vi "generate_simulated_signals.vi"() -> ()   [LabVIEW 2013]
panel:
  out "Mixer signal":dbl[](graph)
  out "Simulated":i16[](graph)
  out "Sine out":fxp<+/-,16,0>[][](array[numeric])
  out "Cosine out":fxp<+/-,16,0>[][](array[numeric])
  out "simulated 2D":i16[][](array[numeric])
  out "simulated 1D":i16[](array[numeric])
  out "sin":fxp<+/-,16,0>[](array[numeric])
  out "cos":fxp<+/-,16,0>[](array[numeric])
  out "Numeric":i32
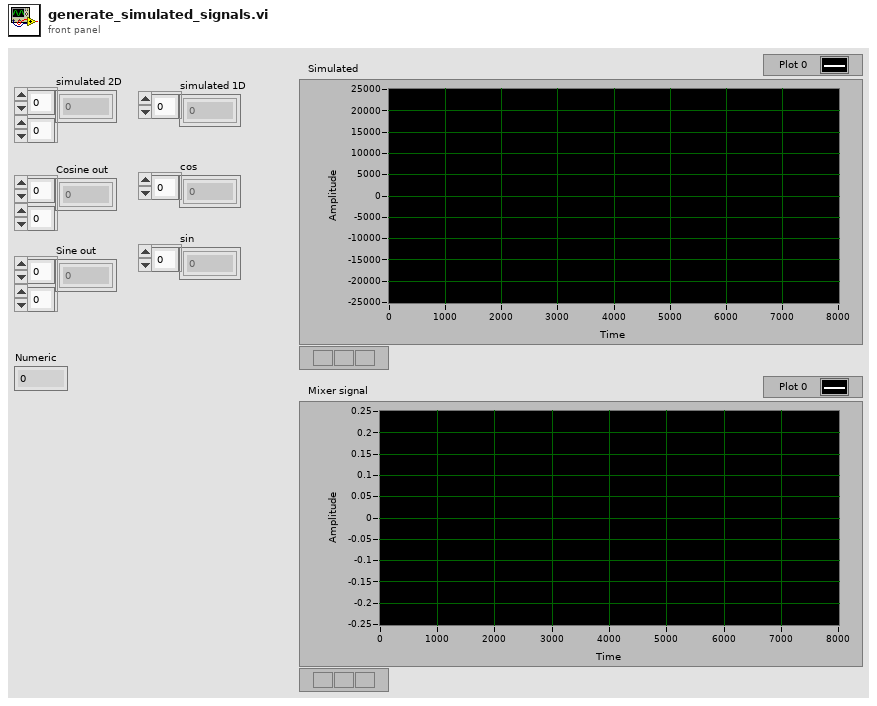
[diagram p1: front panel]
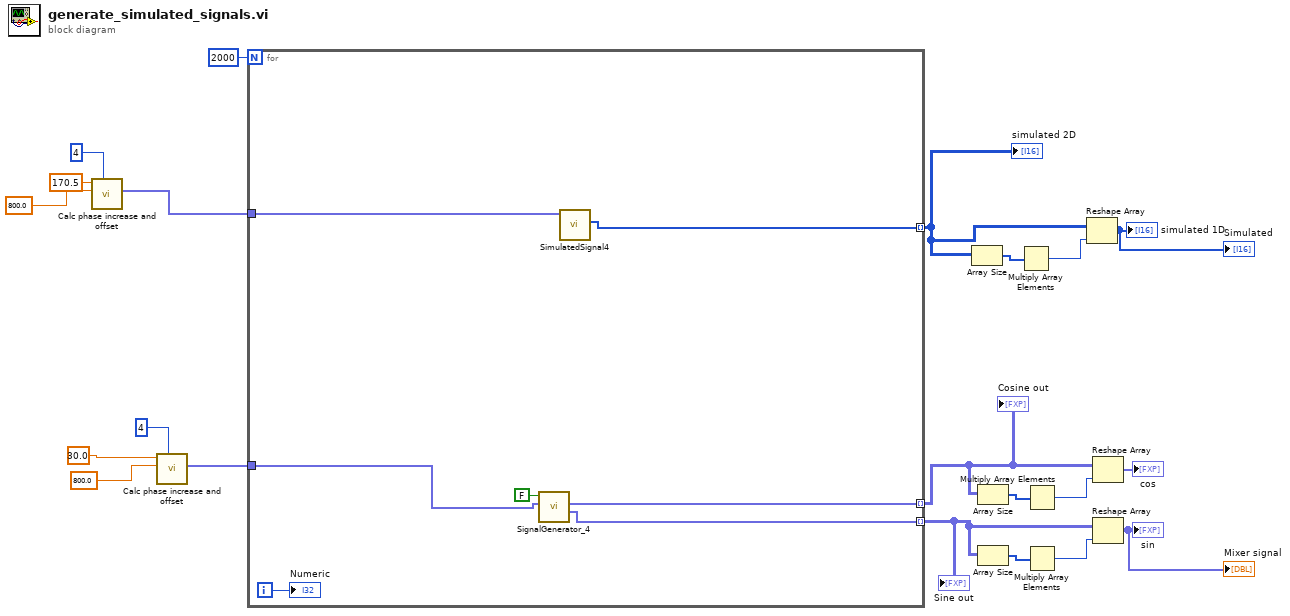
[diagram p0: block diagram]
diagram:
  n1 = call "Calc phase increase and offset.vi"("# of DDS"=4, "fclk (MHz)"=800.0 ("fclk (800MHz)"), "f_generated (MHz)"=170.5) -> ("Phase out"=w3:fxp<+,64,64>[])  [unwired: 6 in, 2 out]
  n2 = call "Calc phase increase and offset.vi"("# of DDS"=4, "fclk (MHz)"=800.0 ("fclk (800MHz)"), "f_generated (MHz)"=30.0) -> ("Phase out"=w15:fxp<+,64,64>[])  [unwired: 6 in, 2 out]
  n3 = for {
    N: 2000 -> [_]
    tunnel: w15 -> [w27]
    tunnel: [w26] -> w11 mode=indexing
    tunnel: [w25] -> w8 mode=indexing
    tunnel: [w23] -> w4 mode=indexing
    tunnel: w3 -> [w22]
    i -> [w24]
    n4 = call "SignalGenerator_4.vi"("Phase"=w27, "reset"=FALSE) -> ("Sine out"=w25:fxp<+/-,16,0>[], "Cosine out"=w26:fxp<+/-,16,0>[])  [unwired: 8 in]
    n5 = call "SimulatedSignal4.vi"("Phase"=w22) -> ("dummy do not use"=w23:i16[])  [unwired: 9 in, 1 out]
    "Numeric" <- w24
  }
  "simulated 2D" <- w4
  "Cosine out" <- w11
  "Sine out" <- w8
  n6 = Array Size(array=w4) -> (size(s)=w5:i32[])
  n7 = Array Size(array=w11) -> (size(s)=w13:i32[])
  n8 = Array Size(array=w8) -> (size(s)=w9:i32[])
  n9 = Multiply Array Elements(1:w5) -> (0:w6:i32)
  n10 = Multiply Array Elements(1:w13) -> (0:w12:i32)
  n11 = Multiply Array Elements(1:w9) -> (0:w10:i32)
  n12 = Reshape Array(w4, w6) -> (→"simulated 1D" →"Simulated":i16[])
  n13 = Reshape Array(w11, w12) -> (→"cos":fxp<+/-,16,0>[])
  n14 = Reshape Array(w8, w10) -> (→"sin" →"Mixer signal":fxp<+/-,16,0>[])
